vi "Receive Dataset.vi"(8 "error in (no error)":errorcluster, 11 "MiniGUI in":refnum<class "MiniGUI.lvclass">) -> (0 "error out":errorcluster, 3 "MiniGUI out":refnum<class "MiniGUI.lvclass">)   [LabVIEW 2019]
uses:
  MiniGUI.lvclass
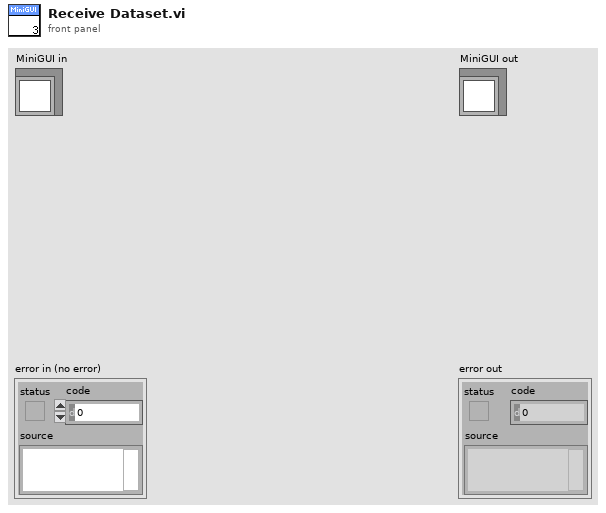
[diagram p1: front panel]
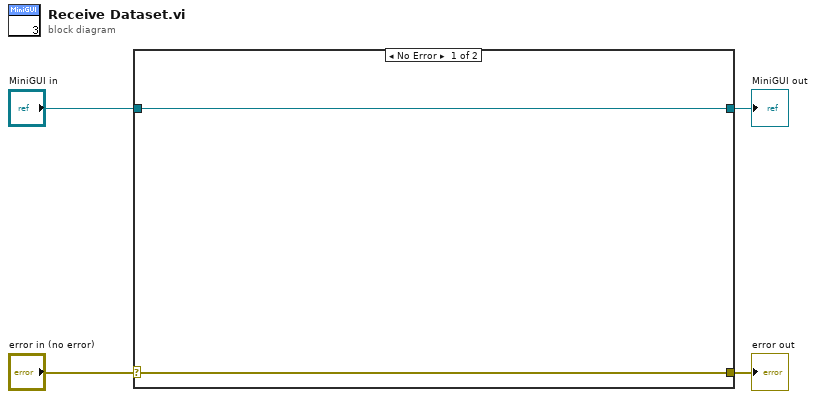
[diagram p0: block diagram]
diagram:
  n1 = case shown="No Error" "error in (no error)" {
    selector: "error in (no error)" -> [w6 w8]
    tunnel: [w6 w8] -> w3
    tunnel: [w5 w7] -> w1
    tunnel: "MiniGUI in" -> [w5 w7]
    frame No Error {
    }
    frame Error {
    }
  }
  "error out" <- w3
  "MiniGUI out" <- w1
